vi "doAction.vi"(8 "error in (no error)":errorcluster, 10 "ContextData":refnum<class "ContextData.lvclass">, 11 "Initialize in":refnum<class "Handle Menu Actions.lvclass">) -> (0 "error out":errorcluster, 2 "ContextData Out":refnum<class "ContextData.lvclass">, 3 "Initialize out":refnum<class "Handle Menu Actions.lvclass">)   [LabVIEW 2020, in "Handle Menu Actions.lvclass"]
uses:
  Handle Menu Actions.lvclass
  ContextData/ContextData.lvclass
  Handle Menu Actions.lvclass/Handle Menu Actions.ctl
  Messages/simonMessages/simonMessages.lvclass
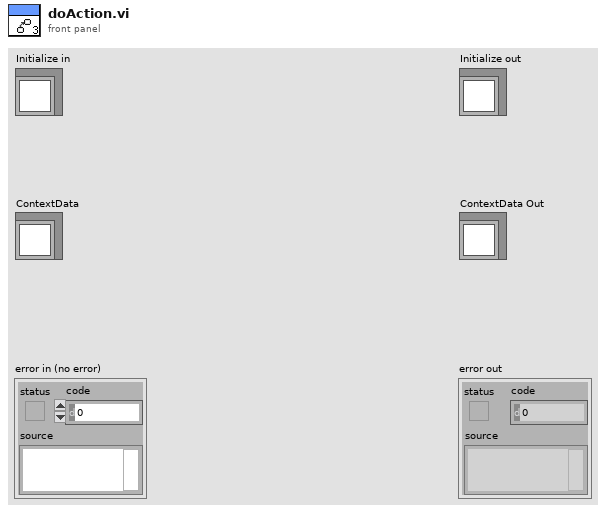
[diagram p1: front panel]
types:
  T1 = cluster{"captionsFile":string, "messageFile":string}
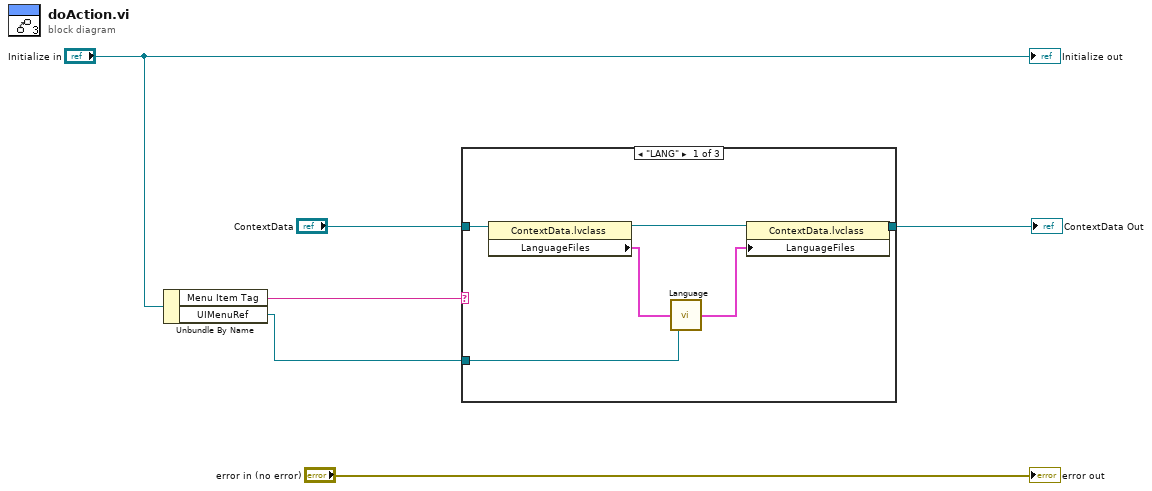
[diagram p0: block diagram]
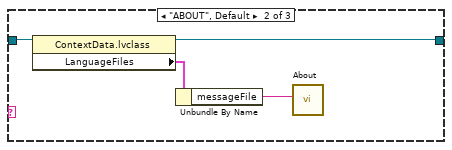
[diagram p2: hidden frame]
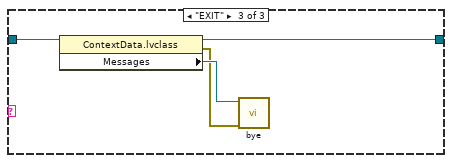
[diagram p3: hidden frame]
diagram:
  n1 = Unbundle By Name("Initialize in") -> ("Menu Item Tag"=w2:string, "UIMenuRef"=w1:refnum<k9>)
  n2 = case shown="\"LANG\"" w2 {
    tunnel: [w12 w16 w20] -> w4
    tunnel: "ContextData" -> [w8 w13 w17]
    tunnel: w1 -> [w7 _ _]
    frame "LANG" {
      n3 = property class="ContextData.lvclass"(reference=w8) -> (reference out=w11:refnum<class "ContextData.lvclass">, "LanguageFiles"=w10:T1)  [unwired: 1 in, 1 out]
      n4 = call "Language.vi"("menu reference"=w7, "LanguageFiles"=w10) -> ("LanguageFiles Out"=w9:T1)  [unwired: 3 in]
      n5 = property class="ContextData.lvclass"(reference=w11, "LanguageFiles"=w9) -> (reference out=w12:refnum<class "ContextData.lvclass">)  [unwired: 1 in, 1 out]
    }
    frame "ABOUT", Default {
      n6 = property class="ContextData.lvclass"(reference=w13) -> (reference out=w16:refnum<class "ContextData.lvclass">, "LanguageFiles"=w15:T1)  [unwired: 1 in, 1 out]
      n7 = Unbundle By Name(w15) -> ("messageFile"=w14:string)
      n8 = call "About.vi"("FileName (without extension)"=w14) -> ()  [unwired: 11 in]
    }
    frame "EXIT" {
      n9 = property class="ContextData.lvclass"(reference=w17) -> (reference out=w20:refnum<class "ContextData.lvclass">, error out=w18:errorcluster, "Messages"=w19:refnum<class "simonMessages.lvclass">)  [unwired: 1 in]
      n10 = call "bye.vi"("error in (no error)"=w18, "simonMessages in"=w19) -> ()  [unwired: 8 in, 2 out]
    }
  }
  "ContextData Out" <- w4
  "error out" <- "error in (no error)"
  "Initialize out" <- "Initialize in"
